vi "arr -- select win.vi"(6 "start index (0)":i32, 9 "z in":cdb[](array[numeric]), 10 "omega in":dbl[](array[numeric]), 11 "cursor window":T3={"left"=2378.60310421286, "right "=2421.6740576496672, "center"=2421.6740576496672, "window"=2421.6740576496672, "cursors"=[], "relative"=0, "absolute"=0, "fixed vertical offset"=2421.6740576496672, "vertical offset"=2421.6740576496672, "skew"=2421.6740576496672, "default window frac"=2421.6740576496672, "kind"=enum."skewed", "skew.left"=2421.6740576496672, "skew.right"=2421.6740576496672, "Plot ref"=refnum, "wing order"=enum."back"}) -> (0 "right index":dbl, 1 "z out":cdb[](array[numeric]), 2 "omega  out":dbl[](array[numeric]), 3 "left index":dbl, 4 "length index":dbl)   [LabVIEW 2020]
uses:
  cursor winow.ctl
  cwin.ctl
  arr action.ctl
panel:
  in  "arr action":T1
  in  "select win":T2={"cen (Hz)"=0.0, "win (Hz)"=0.0, "left (Hz)"=-8.969831627629043, "right (Hz)"=8.26461485679713}
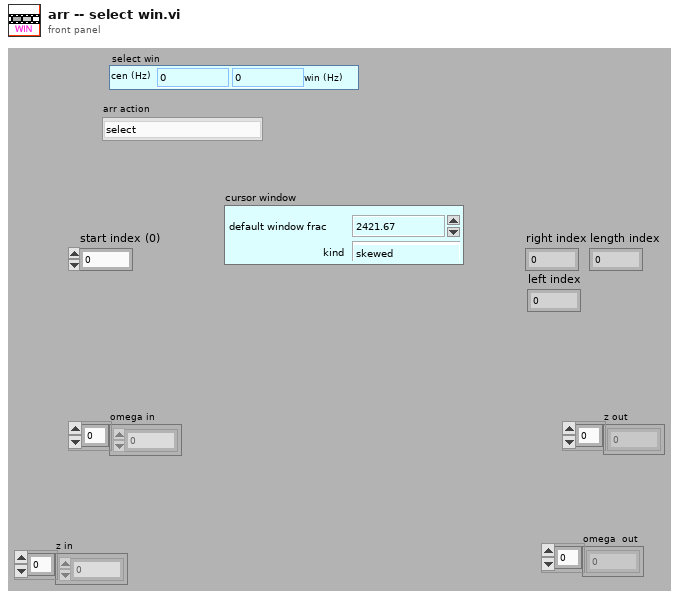
[diagram p1: front panel]
types:
  T1 = typedef "arr action.ctl" = enum16{"select", "remove", "init", "check"}
  T2 = typedef "cwin.ctl" = cluster{"cen (Hz)":dbl, "win (Hz)":dbl, "left (Hz)":dbl, "right (Hz)":dbl}
  T3 = typedef "cursor winow.ctl" = cluster{"left":dbl, "right ":dbl, "center":dbl, "window":dbl, "cursors":i32[], "relative":i32, "absolute":i32, "fixed vertical offset":dbl, "vertical offset":dbl, "skew":dbl, "default window frac":dbl, "kind":enum16{"symmetric", "skewed", "fancy"}, "skew.left":dbl, "skew.right":dbl, "Plot ref":refnum<vi>, "wing order":enum16{"forw", "back"}}
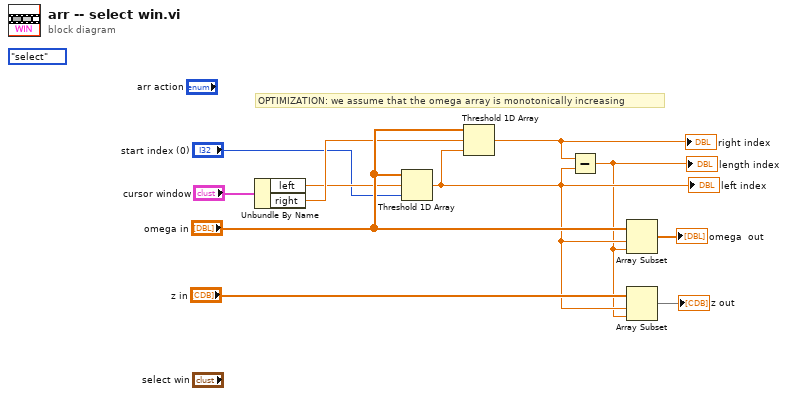
[diagram p0: block diagram]
diagram:
  (unwired) arr_action."select" ("arr action")
  # "OPTIMIZATION: we assume that the omega array is monotonically increasing"
  n1 = Unbundle By Name("cursor window") -> ("left"=w6:dbl, "right"=w7:dbl)
  n2 = Threshold 1D Array(1:"start index (0)", 2:w6, 3:"omega in") -> (0:w2:dbl)
  "left index" <- w2
  n3 = Threshold 1D Array(1:w2, 2:w7, 3:"omega in") -> (0:w11:dbl)
  "right index" <- w11
  n4 = Subtract(x=w11, y=w2) -> (x-y=w1:dbl)
  "length index" <- w1
  n5 = Array Subset(array="omega in", index=w2, length=w1) -> (→"omega  out":dbl[])
  n6 = Array Subset(array="z in", index=w2, length=w1) -> (→"z out":cdb[])
